vi "SSC DAQmx Read (Digital 1D Bool).vi"(0 "DAQmx SSC in":T1[](array[typedef]), 11 "error in":errorcluster) -> (4 "DAQmx SSC out":T1[](array[typedef]), 6 "Per-Task Static State out":bool[][](array[boolean]), 15 "error out":errorcluster)   [LabVIEW 2020]
doc: "Reads one or more Digital states from a task that contains one or more Digital input channels. The data will be ordered based on the SSC order."
uses:
  Pin Map/SSC DAQmx.ctl
  <vilib>/DAQmx/read.llb/DAQmx Read (Digital 1D Bool NChan 1Samp 1Line).vi
  <vilib>/DAQmx/miscellaneous.llb/DAQmx Fill In Error Info.vi
  <resource>/objmgr/daqmx.rc
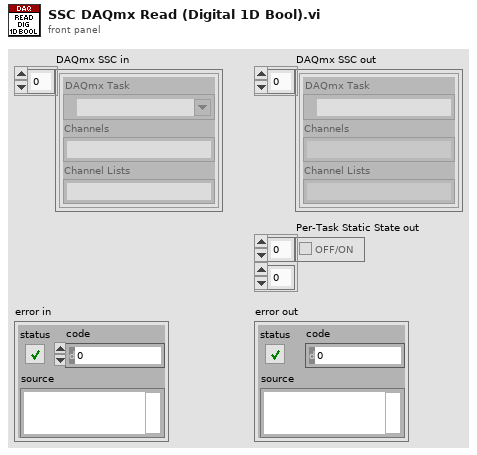
[diagram p1: front panel]
types:
  T1 = typedef "SSC DAQmx.ctl" = cluster{"DAQmx Task ":refnum<k21>, "Channels":string, "Channel Lists":string}
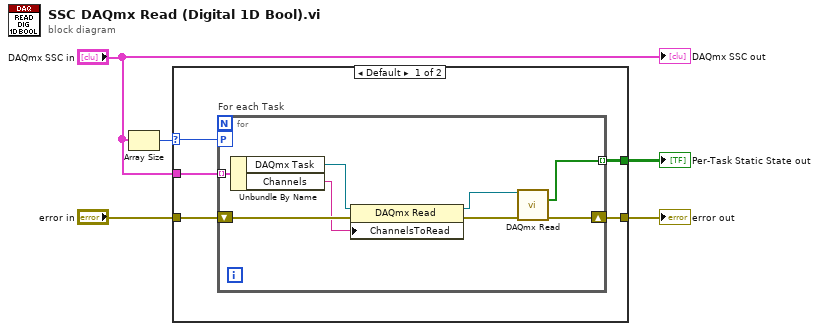
[diagram p0: block diagram]
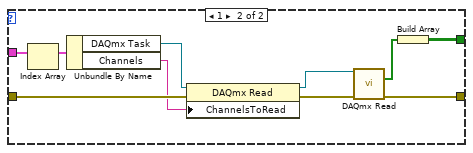
[diagram p2: hidden frame]
diagram:
  n1 = Array Size(array="DAQmx SSC in") -> (size(s)=w5:i32)
  n2 = case shown="Default" w5 {
    selector: w5 -> [w6 _]
    tunnel: "error in" -> [w10 w28]
    tunnel: [w9 w19] -> w1
    tunnel: "DAQmx SSC in" -> [w8 w26]
    tunnel: [w7 w25] -> w4
    frame Default {
      n3 = for "For each Task" {
        tunnel: [w18] -> w9 mode=indexing
        shift-right: [w16] -> w7
        shift-left: w10 -> [w17]
        workers-P: w6 -> [_]
        tunnel: w8 -> [w15] mode=indexing
        n4 = Unbundle By Name(w15) -> ("DAQmx Task"=w12:refnum<k21>, "Channels"=w13:string)
        n5 = property class="DAQmx Read"(reference=w12, error in=w17, "ChannelsToRead"=w13) -> (reference out=w11:refnum<k21>, error out=w14:errorcluster)
        n6 = call-poly <vilib>:"DAQmx Read.vi"("task/channels in"=w11, "error in"=w14) -> ("data"=w18:bool[], "error out"=w16:errorcluster)  [unwired: 11 in, 1 out]
      }
    }
    frame 1 {
      n7 = Index Array(array=w26) -> (element=w20:T1)  [unwired: 1 in]
      n8 = Unbundle By Name(w20) -> ("DAQmx Task"=w22:refnum<k21>, "Channels"=w23:string)
      n9 = property class="DAQmx Read"(reference=w22, error in=w28, "ChannelsToRead"=w23) -> (reference out=w21:refnum<k21>, error out=w24:errorcluster)
      n10 = call-poly <vilib>:"DAQmx Read.vi"("task/channels in"=w21, "error in"=w24) -> ("data"=w27:bool[], "error out"=w25:errorcluster)  [unwired: 11 in, 1 out]
      n11 = Build Array(w27) -> (w19:bool[][])
    }
  }
  "Per-Task Static State out" <- w1
  "error out" <- w4
  "DAQmx SSC out" <- "DAQmx SSC in"
